vi "Channel Name to Variables.vi"(11 "Channel Name":string) -> (1 "hostname":string, 2 "Variable Name":string, 3 "Protocol":T1)   [LabVIEW 2013, in "Scan Engine editor node.lvclass"]
uses:
  Scan Engine editor node.lvclass
  configuration/Protocol.ctl
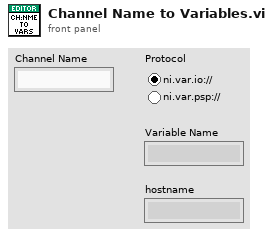
[diagram p1: front panel]
types:
  T1 = typedef "Scan Engine editor node.lvclass/Protocol.ctl" = enum32{"ni.var.io://", "ni.var.psp://"}
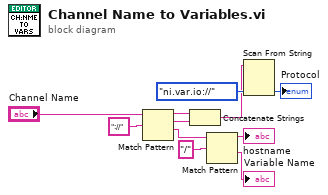
[diagram p0: block diagram]
diagram:
  n1 = Match Pattern(string="Channel Name", regular expression="://") -> (before substring=w3:string, match substring=w2:string, after substring=w1:string)  [unwired: 1 in, 1 out]
  n2 = Concatenate Strings(w3, w2) -> (w4:string)
  n3 = Match Pattern(string=w1, regular expression="/") -> (before substring=→"hostname":string, after substring=→"Variable Name":string)  [unwired: 1 in, 2 out]
  n4 = Scan From String(input string=w4, default 1=Protocol."ni.var.io://" ("URL")) -> (output 1=→"Protocol":T1)  [unwired: 3 in, 3 out]
